vi "Move Absolute SubVi.vi"(2 "error in":errorcluster, 3 "Vel and Acc":cluster{"vel":dbl, "Acc":dbl}, 4 "Absolute Movement":cluster{"X Position":dbl, "Y Position":dbl}[](array[cluster]), 5 "reference in":refnum<k24>) -> (0 "error out":errorcluster, 1 "reference out":refnum<k24>)   [LabVIEW 2017]
uses:
  Newport.XPS.CommandInterface
  Absolute Move Enum.ctl
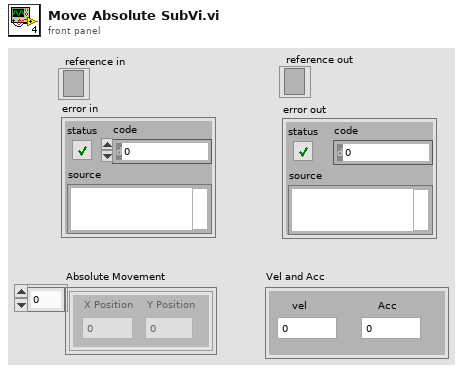
[diagram p1: front panel]
types:
  T1 = typedef "Absolute Move Enum.ctl" = enum16{"Change Velocity", "Move Position", "Stop Command"}
  T2 = cluster{"Absolute Movement[0]":cluster{"X Position":dbl, "Y Position":dbl}, "Absolute Movement[1]":cluster{"X Position":dbl, "Y Position":dbl}, "Absolute Movement[2]":cluster{"X Position":dbl, "Y Position":dbl}, "Absolute Movement[3]":cluster{"X Position":dbl, "Y Position":dbl}, "Absolute Movement[4]":cluster{"X Position":dbl, "Y Position":dbl}, "Absolute Movement[5]":cluster{"X Position":dbl, "Y Position":dbl}, "Absolute Movement[6]":cluster{"X Position":dbl, "Y Position":dbl}, "Absolute Movement[7]":cluster{"X Position":dbl, "Y Position":dbl}, "Absolute Movement[8]":cluster{"X Position":dbl, "Y Position":dbl}}
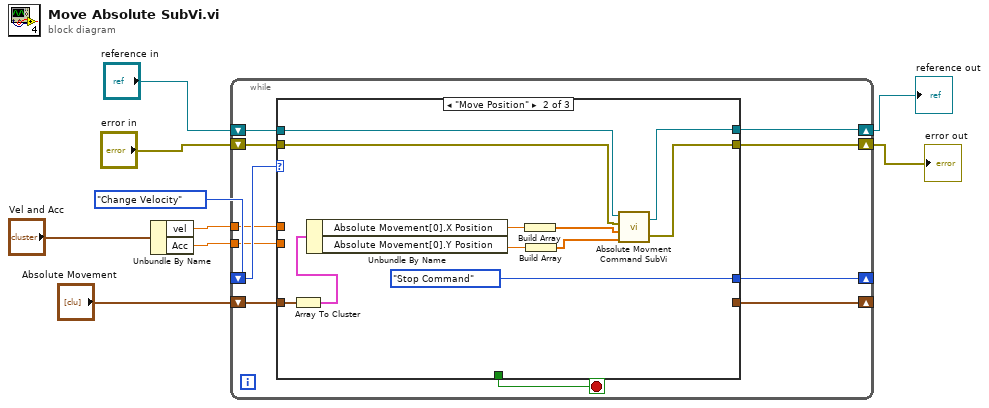
[diagram p0: block diagram]
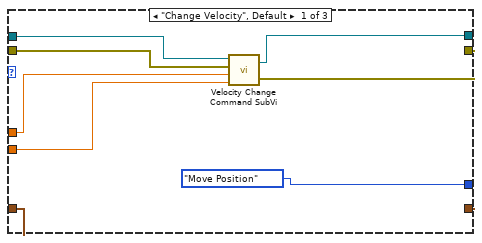
[diagram p2: hidden frame]
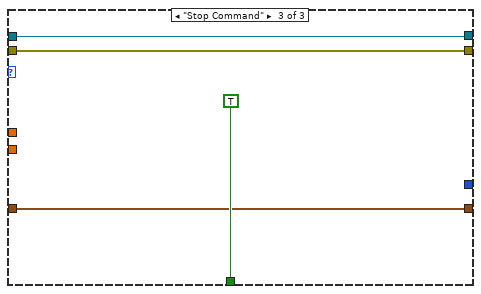
[diagram p3: hidden frame]
diagram:
  n1 = Unbundle By Name("Vel and Acc") -> ("vel"=w2:dbl, "Acc"=w1:dbl)
  n2 = while {
    shift-right: [w20] -> _
    shift-left: Absolute_Move_Enum."Change Velocity" -> [w17]
    shift-right: [w14] -> w5
    shift-left: "error in" -> [w18]
    shift-right: [w15] -> w6
    shift-left: "reference in" -> [w19]
    shift-right: [w12] -> _
    shift-left: "Absolute Movement" -> [w13]
    tunnel: w2 -> [w11]
    tunnel: w1 -> [w10]
    stop <- w16 stop-if-true
    n3 = case shown="\"Move Position\"" w17 {
      tunnel: [Absolute_Move_Enum."Move Position" Absolute_Move_Enum."Stop Command" _] -> w20
      tunnel: w19 -> [w27 w32 w42]
      tunnel: w18 -> [w26 w31 w41]
      tunnel: [w23 w30 w42] -> w15
      tunnel: [w22 w29 w41] -> w14
      tunnel: [_ _ TRUE] -> w16
      tunnel: w13 -> [w28 w36 w40]
      tunnel: [w28 _ w40] -> w12
      tunnel: w11 -> [w25 _ _]
      tunnel: w10 -> [w24 _ _]
      frame "Change Velocity", Default {
        n4 = call "Velocity Change Command SubVi.vi"("Acceleration"=w24, "Velocity"=w25, "error in"=w26, "reference in"=w27) -> ("error out"=w22:errorcluster, "reference out"=w23:refnum<k24>)
      }
      frame "Move Position" {
        n5 = Array To Cluster(array=w36) -> (cluster=w37:T2)
        n6 = Unbundle By Name(w37) -> ("Absolute Movement[0].X Position"=w38:dbl, "Absolute Movement[0].Y Position"=w39:dbl)
        n7 = Build Array(w38) -> (w34:dbl[])
        n8 = Build Array(w39) -> (w33:dbl[])
        n9 = call "Absolute Movment Command SubVi.vi"("TargetPosition Y"=w33, "TargetPosition X"=w34, "error in"=w31, "reference in"=w32) -> ("error out"=w29:errorcluster, "reference out"=w30:refnum<k24>)
      }
      frame "Stop Command" {
      }
    }
  }
  "reference out" <- w6
  "error out" <- w5
